vi "Position Update.vi"(2 "Y position in":dbl, 3 "X position in":dbl, 4 "Distance":dbl, 5 "Heading":dbl) -> (0 "Y position":dbl, 1 "X position":dbl)   [LabVIEW 2019]
panel:
  in  "Cluster":T1
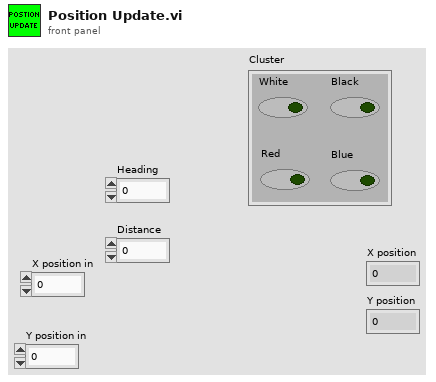
[diagram p1: front panel]
types:
  T1 = cluster{"White":bool, "Black":bool, "Red":bool, "Blue":bool}
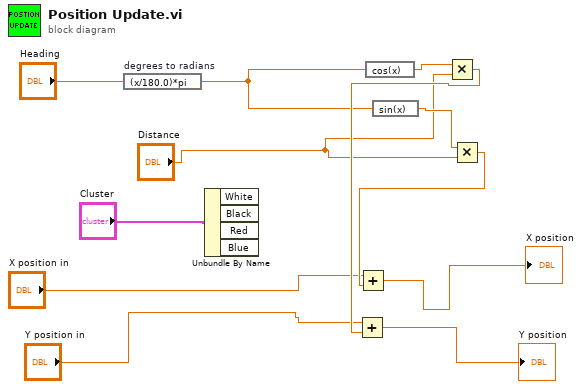
[diagram p0: block diagram]
diagram:
  n1 = expression code="(x/180.0)*pi" "degrees to radians"("Heading") -> (w5:dbl)
  n2 = Unbundle By Name("Cluster") -> ()  [unwired: 4 out]
  n3 = expression code="cos(x)"(w5) -> (w11:dbl)
  n4 = expression code="sin(x)"(w5) -> (w12:dbl)
  n5 = Multiply(x=w11, y="Distance") -> (x*y=w9:dbl)
  n6 = Add(x="Y position in", y=w9) -> (x+y=→"Y position":dbl)
  n7 = Multiply(x=w12, y="Distance") -> (x*y=w10:dbl)
  n8 = Add(x="X position in", y=w10) -> (x+y=→"X position":dbl)
